vi "macro_NumCmd_Recv_Chassis.vi"() -> ()   [LabVIEW 2019, in "Trajectory_Library.lvlib"]
uses:
  VI/BoolCmd_Recv_Internal.vi
  VI/BoolCmd_ObtainQueue.vi
  Trajectory_Library.lvlib
  TypeDef/CHASSIS_SPEEDS.ctl
panel:
  out "Chassis Speeds-demand":T1 {"vOmega" format="%10.3f"; "vY" format="%10.3f"; "vX" format="%10.3f"}
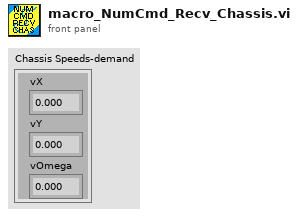
[diagram p1: front panel]
types:
  T1 = typedef "Trajectory_Library.lvlib/CHASSIS_SPEEDS.ctl" = cluster{"vX":dbl, "vY":dbl, "vOmega":dbl}
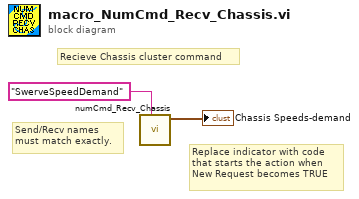
[diagram p0: block diagram]
diagram:
  # "Send/Recv names\nmust match exactly."
  # "Replace indicator with code\nthat starts the action when \nNew Request becomes TRUE"
  # "Recieve Chassis cluster command"
  n1 = call "numCmd_Recv_Chassis.vi"("Command Name"="SwerveSpeedDemand") -> ("Chassis Speeds"=→"Chassis Speeds-demand":T1)  [unwired: 8 in, 2 out]
